vi "Store Data Core.vi"(8 "Error In":errorcluster, 10 "LHW-DataCollection":refnum<class "LHW-DataCollection.lvclass">, 11 "LHW-TDMS-Storage-Actor in":refnum<class "LHW-TDMS-Storage-Actor.lvclass">) -> (0 "Error Out":errorcluster, 3 "LHW-TDMS-Storage-Actor out":refnum<class "LHW-TDMS-Storage-Actor.lvclass">)   [LabVIEW 2014, in "LHW-TDMS-Storage.lvlib" / "LHW-TDMS-Storage-Actor.lvclass"]
doc: "Store received data."
uses:
  LHW-TDMS-Storage-Actor.lvclass
  Classes/LHW-Data/LHW-DataCollection/LHW-DataCollection.lvclass
  Classes/LHW-Data/LHW-Data/LHW-Data.lvclass
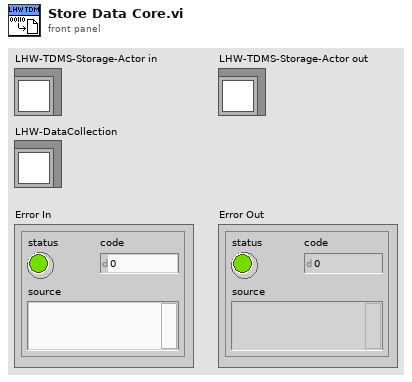
[diagram p1: front panel]
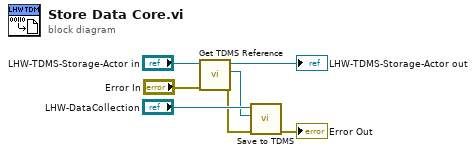
[diagram p0: block diagram]
diagram:
  n1 = call "Get TDMS Reference.vi"("Error In"="Error In", "LHW-TDMS-Storage-Actor in"="LHW-TDMS-Storage-Actor in") -> ("Error Out"=w2:errorcluster, "TDMS Ref"=w3:refnum<k34>, "LHW-TDMS-Storage-Actor out"=→"LHW-TDMS-Storage-Actor out":refnum<class "LHW-TDMS-Storage-Actor.lvclass">)  [unwired: 7 in]
  n2 = call "Save to TDMS.vi"("Error In"=w2, "TDMS Ref"=w3, "LHW-Data in"="LHW-DataCollection") -> ("Error Out"=→"Error Out":errorcluster)  [unwired: 7 in, 1 out]
